vi "PID Internals_CMD.vi"(0 "Run PI?":bool, 1 "LimitCluster":T1, 2 "FFcluster":cluster{"FF_m":dbl, "FF_b":dbl}, 3 "PI Far->Close":dbl[][](array[numeric]), 5 "SP":dbl, 7 "Error":dbl, 9 "SPZero":bool, 12 "IndirectMin?":bool, 13 "Stop CMD":dbl, 14 "CmdChanged":bool) -> (4 "SlewIndex":dbl, 8 "Output":dbl)   [LabVIEW 2019]
uses:
  <vilib>/addons/control/pid/pid.llb/PID Output Rate Limiter (DBL).vi
  <vilib>/addons/control/pid/NI_PID_pid.lvlib
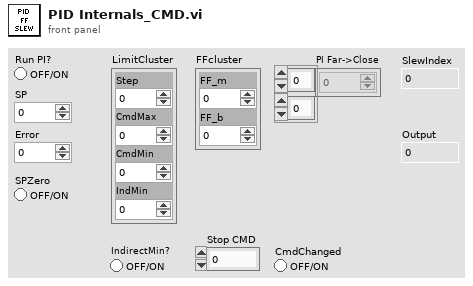
[diagram p1: front panel]
types:
  T1 = cluster{"Step":dbl, "CmdMax":dbl, "CmdMin":dbl, "IndMin":dbl}
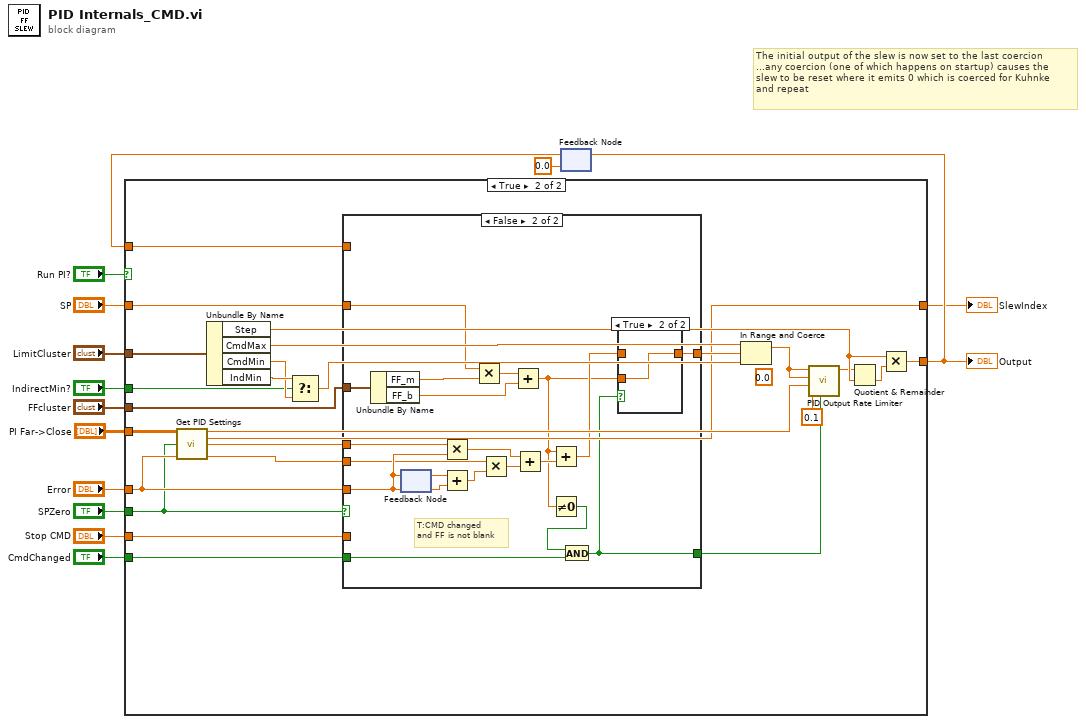
[diagram p0: block diagram]
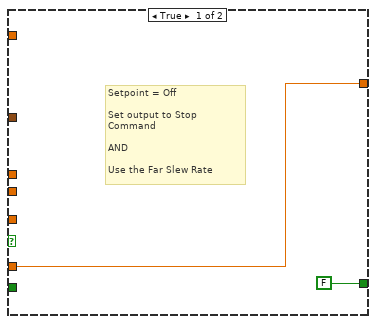
[diagram p3: hidden frame]
diagram:
  # "The initial output of the slew is now set to the last coercion\n...any coercion (one of which happens on startup) causes the\nslew to be reset where it emits 0 which is coerced for Kuhnke\nand repeat"
  n1 = feedback #1(0.0 ("SP")) -> (w13:dbl)
  n2 = case shown="True" "Run PI?" {
    tunnel: [w15 w19] -> w6
    tunnel: "SP" -> [w15 w41]
    tunnel: "Error" -> [_ w27]
    tunnel: "FFcluster" -> [_ w40]
    tunnel: "LimitCluster" -> [_ w38]
    tunnel: "SPZero" -> [_ w26]
    tunnel: w13 -> [_ w39]
    tunnel: [w15 w16] -> w5
    tunnel: "IndirectMin?" -> [_ w34]
    tunnel: "Stop CMD" -> [_ w30]
    tunnel: "CmdChanged" -> [_ w29]
    tunnel: "PI Far->Close" -> [_ w28]
    frame False {
    }
    frame True {
      (unwired) 0.0 ("initial output")
      n3 = call "Get PID Settings.vi"("PI Far->Close"=w28, "SPzero"=w26, "Error"=w27) -> ("Slew"=w25:dbl, "SlewIndex"=w16:dbl, "Kp"=w24:dbl, "Ki"=w23:dbl)  [unwired: 9 in]
      n4 = Unbundle By Name(w38) -> ("Step"=w33:dbl, "CmdMax"=w32:dbl, "CmdMin"=w35:dbl, "IndMin"=w36:dbl)
      n5 = Select(t=w36, s=w34, f=w35) -> (s? t:f=w31:dbl)
      n6 = case shown="False" w26 {
        tunnel: w41 -> [_ w60]
        tunnel: w27 -> [_ w58]
        tunnel: w40 -> [_ w54]
        tunnel: w39 -> [_ _]
        tunnel: w24 -> [_ w51]
        tunnel: w23 -> [_ w50]
        tunnel: [w43 w48] -> w37
        tunnel: w30 -> [w43 _]
        tunnel: w29 -> [_ w47]
        tunnel: [FALSE w44] -> w18
        frame True {
          # "Setpoint = Off\n\nSet output to Stop Command\n\nAND\n\nUse the Far Slew Rate"
        }
        frame False {
          # "T:CMD changed\nand FF is not blank"
          n7 = Unbundle By Name(w54) -> ("FF_m"=w53:dbl, "FF_b"=w52:dbl)
          n8 = feedback #2(w58) -> (w59:dbl)
          n9 = feedback-in #2(w58) -> ()
          n10 = Multiply(x=w51, y=w58) -> (x*y=w56:dbl)
          n11 = Add(x=w59, y=w58) -> (x+y=w55:dbl)
          n12 = Multiply(x=w60, y=w53) -> (x*y=w62:dbl)
          n13 = Multiply(x=w50, y=w55) -> (x*y=w57:dbl)
          n14 = Add(x=w62, y=w52) -> (x+y=w46:dbl)
          n15 = Add(x=w56, y=w57) -> (x+y=w61:dbl)
          n16 = Add(x=w46, y=w61) -> (x+y=w49:dbl)
          n17 = Not Equal To 0?(x=w46) -> (x != 0?=w45:bool)
          n18 = And(x=w45, y=w47) -> (x .and. y?=w44:bool)
          n19 = case shown="True" w44 {
            tunnel: w49 -> [w63 _]
            tunnel: [w63 w64] -> w48
            tunnel: w46 -> [_ w64]
            frame False {
            }
            frame True {
            }
          }
        }
      }
      n20 = In Range and Coerce(upper limit=w32, x=w37, lower limit=w31) -> (coerced(x)=w17:dbl)  [unwired: 1 out]
      n21 = call-poly <vilib>:"PID Output Rate Limiter.vi"("reinitialize? (F)"=w18, "dt (s)"=0.1, "output rate (EGU/min)"=w25, "initial output"=w17, "input (controller output)"=w17) -> ("output"=w22:dbl)  [unwired: 3 in, 1 out]
      n22 = Quotient & Remainder(x=w22, y=w33) -> (floor(x/y)=w21:dbl)  [unwired: 1 out]
      n23 = Multiply(x=w33, y=w21) -> (x*y=w19:dbl)
    }
  }
  "Output" <- w6
  "SlewIndex" <- w5
  n24 = feedback-in #1(w6) -> ()
